vi "estimate_AT_and_E0.vi"(3 "EMFs":dbl[](array[numeric]), 4 "HCl Concentration":dbl, 5 "k":dbl, 6 "Sample Mass":dbl, 7 "Total HCl masses":dbl[](array[numeric])) -> (0 "AT Estimate":dbl, 1 "E0 Estimate":dbl)   [LabVIEW 2010]
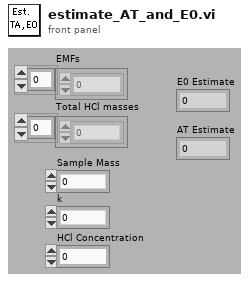
[diagram p1: front panel]
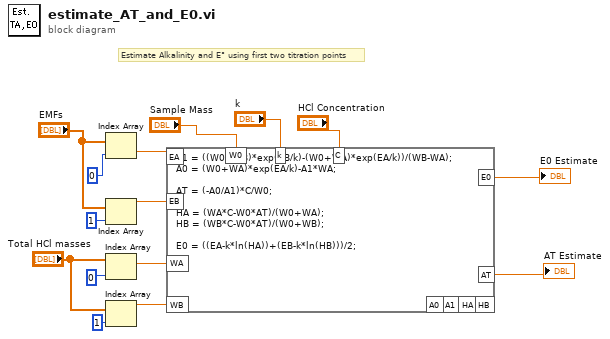
[diagram p0: block diagram]
diagram:
  # "Estimate Alkalinity and E° using first two titration points"
  n1 = Index Array(array="EMFs", index=0 ("Index")) -> (element=w11:dbl)
  n2 = Index Array(array="EMFs", index=1 ("Index")) -> (element=w10:dbl)
  n3 = Index Array(array="Total HCl masses", index=0 ("Index")) -> (element=w9:dbl)
  n4 = Index Array(array="Total HCl masses", index=1 ("Index")) -> (element=w8:dbl)
  n5 = formula code="A1 = ((W0+WB)*exp(EB/k)-(W0+WA)*exp(EA/k))/(WB-WA);\nA0 = (W0+WA)*exp(EA/k)-A1*WA;\n\nAT = (-A0/A1)*C/W0;\n\nHA = (WA*C-W0*AT)/(W0+WA);\nHB = (WB*C-W0*AT)/(W0+WB);\n\nE0 = ((EA-k*ln(HA))+(EB-k*ln(HB)))/2;"("EA"=w11, "EB"=w10, "W0"="Sample Mass", "WB"=w8, "WA"=w9, "k"="k", "C"="HCl Concentration") -> ("AT"=→"AT Estimate":dbl, "E0"=→"E0 Estimate":dbl)  [unwired: 4 out]
